vi "Read TC State Machine Setups.vi"(4 "Error In":errorcluster, 5 "Reload?":bool, 6 "Instance Name":T2, 7 "DB_ADO in":refnum<class "Config Data_DB_ADO.lvclass">) -> (0 "Error Out":errorcluster, 2 "TC Parameters":T1, 3 "DB_ADO out":refnum<class "Config Data_DB_ADO.lvclass">)   [LabVIEW 2020, in "Config Data.lvlib" / "Config Data_DB_ADO.lvclass"]
uses:
  Config Data_DB_ADO.lvclass
  toolbox/ADO Database Drivers/ADO Database Drivers.lvlib
  Config Data_DB.lvclass
  C:/Users/Fred Guo/Desktop/Release 19/_libraries/Config Data/DB/Config Data_DB.lvclass
  C:/Users/Fred Guo/Desktop/Release 19/_libraries/Config Data/Config Data.lvclass
  C:/Users/Fred Guo/Desktop/Release 19/_libraries/Config Data/DB/ADO/Config Data_DB_ADO.lvclass
  Startup Processes/_typedefs/Subpanel Names.ctl
  Startup Processes/Startup Processes.lvlib
  Startup Processes/_typedefs/TC Setup Parameters.ctl
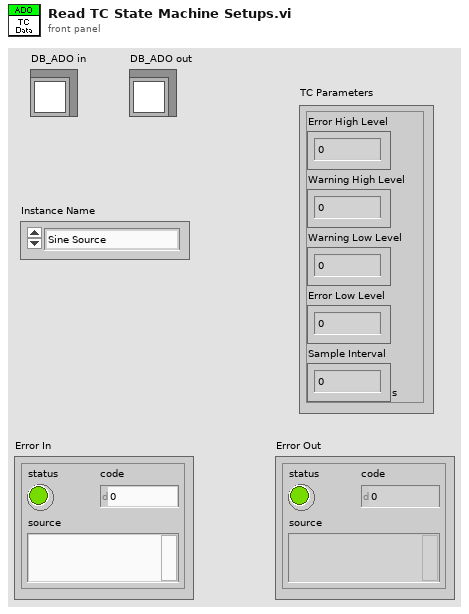
[diagram p1: front panel]
types:
  T1 = typedef "Startup Processes.lvlib/TC Setup Parameters.ctl" = cluster{"Error High Level":dbl, "Warning High Level":dbl, "Warning Low Level":dbl, "Error Low Level":dbl, "Sample Interval":dbl[unit]}
  T2 = typedef "Startup Processes.lvlib/Subpanel Names.ctl" = enum16{"Sine Source", "Ramp Source", "Hen House TC", "Dog House TC", "Out House TC"}
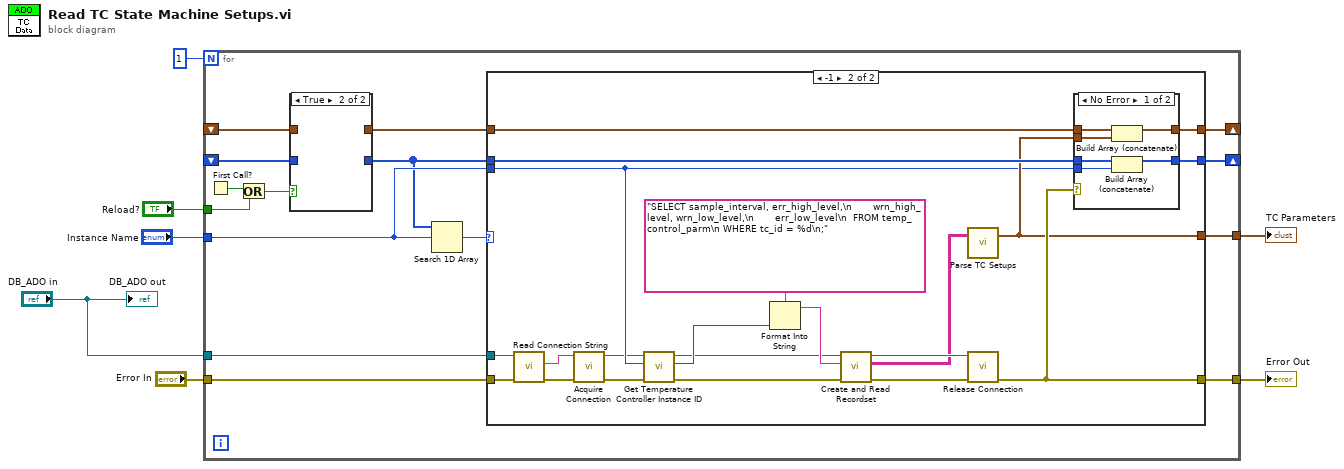
[diagram p0: block diagram]
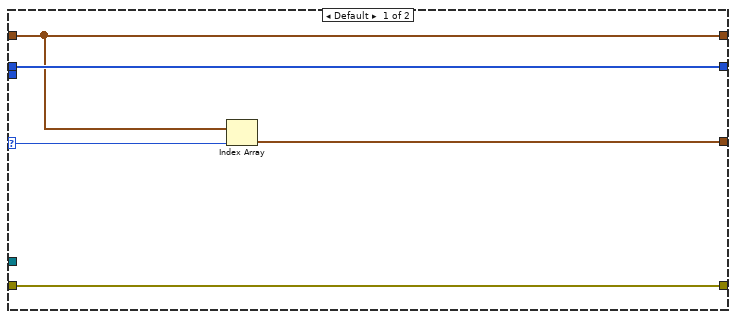
[diagram p3: hidden frame]
diagram:
  n1 = for {
    N: 1 -> [_]
    tunnel: "Error In" -> [w22]
    tunnel: [w21] -> w3
    shift-right: [w20] -> _
    shift-left: _ -> [w16]
    shift-right: [w19] -> _
    shift-left: _ -> [w15]
    tunnel: "Instance Name" -> [w17]
    tunnel: [w12] -> w2
    tunnel: "DB_ADO in" -> [w11]
    tunnel: "Reload?" -> [w8]
    n2 = First Call?() -> (First Call?: T/F=w9:bool)
    n3 = Or(x=w9, y=w8) -> (x .or. y?=w10:bool)
    n4 = case shown="True" w10 {
      tunnel: w16 -> [w24 _]
      tunnel: w15 -> [w23 _]
      tunnel: [w24 _] -> w14
      tunnel: [w23 _] -> w13
      frame False {
      }
      frame True {
      }
    }
    n5 = Search 1D Array(1D array=w13, element=w17) -> (index of element=w18:i32)  [unwired: 1 in]
    n6 = case shown="-1" w18 {
      selector: w18 -> [w27 _]
      tunnel: w22 -> [w29 w31]
      tunnel: [w29 w45] -> w21
      tunnel: w14 -> [w26 w44]
      tunnel: [w26 w42] -> w20
      tunnel: [w28 w41] -> w19
      tunnel: w13 -> [w28 w43]
      tunnel: w17 -> [_ w38]
      tunnel: [w25 w40] -> w12
      tunnel: w11 -> [_ w30]
      frame Default {
        n7 = Index Array(array=w26, index=w27) -> (element=w25:T1)
      }
      frame -1 {
        n8 = call "Read Connection String.vi"("Error In"=w31, "DB In"=w30) -> ("Error Out"=w33:errorcluster, "Connection String"=w32:string)  [unwired: 3 in, 1 out]
        n9 = call "Acquire Connection.vi"("error in (no error)"=w33, "Connection String"=w32) -> ("error out"=w35:errorcluster, "Connection"=w34:refnum<k7>)  [unwired: 3 in, 1 out]
        n10 = call "Get Temperature Controller Instance ID.vi"("error in (no error)"=w35, "Instance Name"=w38, "Connection In"=w34) -> ("error out"=w39:errorcluster, "tc_id"=w37:i32, "Connection Out"=w36:refnum<k7>)  [unwired: 2 in]
        n11 = Format Into String(format string="SELECT sample_interval, err_high_level,\n       wrn_high_level, wrn_low_level,\n       err_low_level\n  FROM temp_control_parm\n WHERE tc_id = %d\n;", w37) -> (resulting string=w47:string)  [unwired: 2 in, 1 out]
        n12 = call "Create and Read Recordset.vi"("error in (no error)"=w39, "Source"=w47, "Connection In"=w36) -> ("error out"=w50:errorcluster, "DB Data"=w48:string[][], "Connection Out"=w49:refnum<k7>)  [unwired: 2 in, 2 out]
        n13 = call "Parse TC Setups.vi"("DB Data"=w48) -> ("TC Parameters"=w40:T1)  [unwired: 2 in]
        n14 = call "Release Connection.vi"("error in"=w50, "Connection"=w49) -> ("error out"=w45:errorcluster)  [unwired: 5 in]
        n15 = case shown="No Error" w45 {
          tunnel: w44 -> [w56 w58]
          tunnel: w43 -> [w53 w57]
          tunnel: [w54 w58] -> w42
          tunnel: [w52 w57] -> w41
          tunnel: w40 -> [w55 _]
          tunnel: w38 -> [w51 _]
          frame No Error {
            n16 = Build Array (concatenate)(w56, w55) -> (w54:T1[])
            n17 = Build Array (concatenate)(w53, w51) -> (w52:T2[])
          }
          frame Error {
          }
        }
      }
    }
  }
  "Error Out" <- w3
  "TC Parameters" <- w2
  "DB_ADO out" <- "DB_ADO in"
